vi "File5.vi"() -> ()   [LabVIEW 2019]
uses:
  Control 3.ctl
  Control 1.ctl
  Control 2.ctl
panel:
  in  "Velikost okna":dbl(ring)=0.25 items=["100ms"=0.1, "250ms"=0.25, "500ms"=0.5, "1s"=1.0]
  out "XY Graph":cluster{"Array":dbl[], "Y":dbl[]}(graph)
  in  "Pocet vzorku":i32
  in  "Rychlost ubihani 2":T1=0.1 step=5e-05
  in  "Cas necitlivosti 2":dbl
  in  "Fvz 2":T2
  in  "Offset 2":dbl format="%0.2p"
  in  "Ubihani 2":bool
  in  "Frekvence 2":dbl=10.0 format="%0.2p"
  in  "Amplituda sumu 2":T3
  in  "Amplituda 2":dbl=1.0 format="%0.2p"
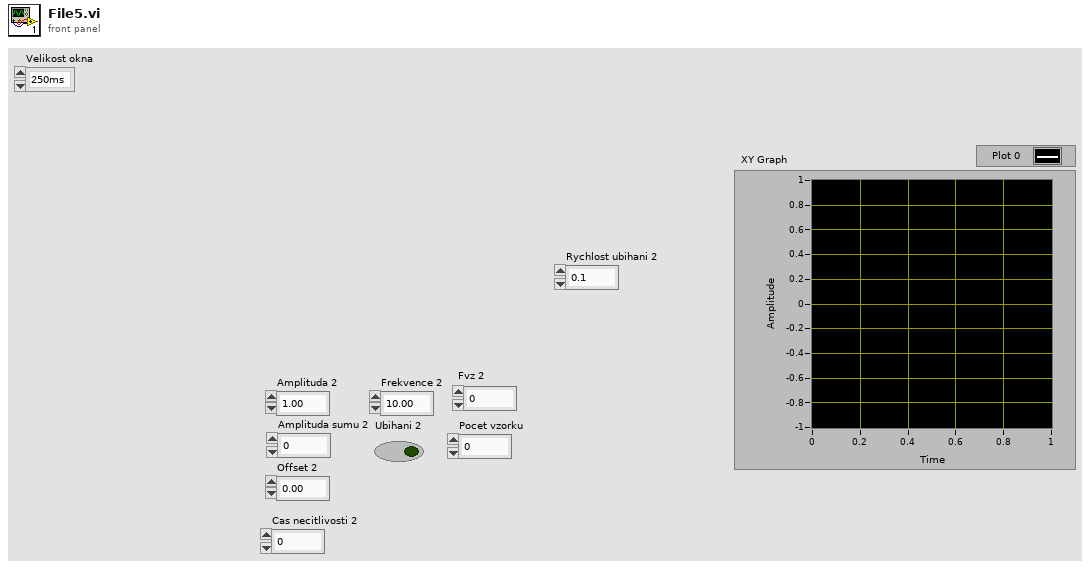
[diagram p1: front panel]
types:
  T1 = typedef "Control 2.ctl" = dbl
  T2 = typedef "Control 1.ctl" = dbl
  T3 = typedef "Control 3.ctl" = dbl
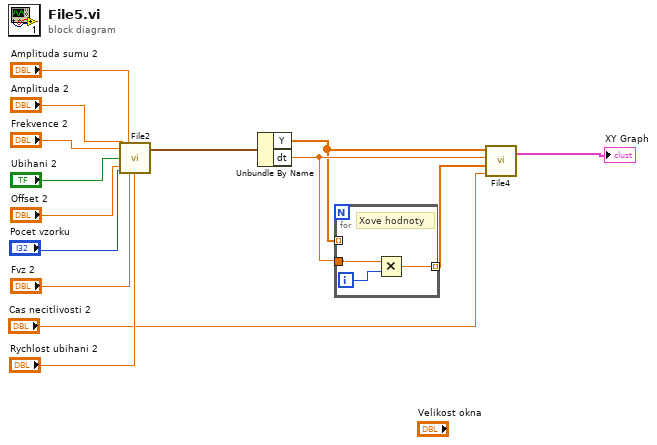
[diagram p0: block diagram]
diagram:
  n1 = call "File2.vi"("Amplituda"="Amplituda 2", "Amplituda sumu"="Amplituda sumu 2", "Rychlost ubihani"="Rychlost ubihani 2", "Frekvence"="Frekvence 2", "Ubihani"="Ubihani 2", "Offset"="Offset 2", "Pocet vzorku"="Pocet vzorku", "Fvz"="Fvz 2") -> ("Output"=w8:waveform(dbl))  [unwired: 6 in, 1 out]
  n2 = Unbundle By Name(w8) -> ("Y"=w2:dbl[], "dt"=w6:dbl)
  n3 = for {
    tunnel: w6 -> [w17]
    tunnel: [w15] -> w5 mode=indexing
    tunnel: w2 -> [_] mode=indexing
    i -> [w16]
    # "Xove hodnoty"
    n4 = Multiply(x=w17, y=w16) -> (x*y=w15:dbl)
  }
  n5 = call "File4.vi"("Pocet ignorovanych vzorku"="Cas necitlivosti 2", "X"=w5, "dt"=w6, "Y"=w2) -> ("XY Graph"=→"XY Graph":cluster{"Array":dbl[], "Y":dbl[]})  [unwired: 1 out]
